vi "Get Pressure.vi"(6 "Channel":i32, 8 "error in (no error)":errorcluster, 11 "Instrument.Cryostat in":refnum<class "Instrument.Cryostat.lvclass">) -> (0 "error out":errorcluster, 1 "Status":string, 2 "Pressure (mbar)":dbl, 3 "Instrument.Cryostat out":refnum<class "Instrument.Cryostat.lvclass">)   [LabVIEW 2019, in "Instrument.Cryostat.lvclass"]
uses:
  Instrument.Cryostat.lvclass
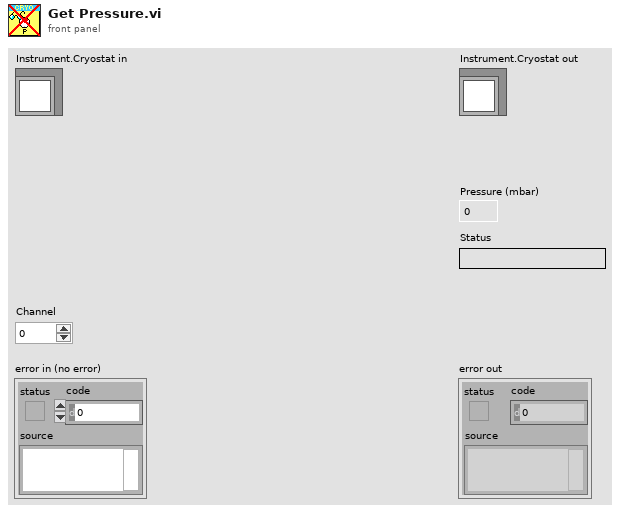
[diagram p1: front panel]
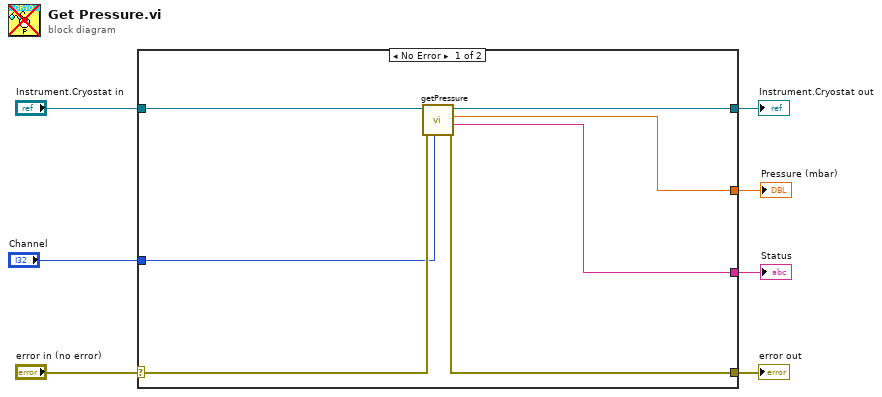
[diagram p0: block diagram]
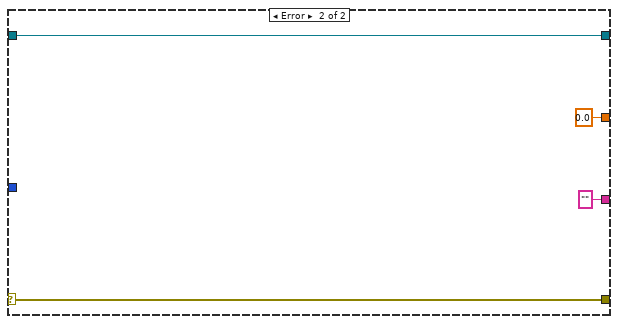
[diagram p2: hidden frame]
diagram:
  n1 = case shown="No Error" "error in (no error)" {
    selector: "error in (no error)" -> [w12 w18]
    tunnel: [w11 w18] -> w6
    tunnel: [w14 w17] -> w4
    tunnel: "Instrument.Cryostat in" -> [w13 w17]
    tunnel: [w10 "" ("Status")] -> w3
    tunnel: [w9 0.0 ("Pressure (mbar)")] -> w2
    tunnel: "Channel" -> [w8 _]
    frame No Error {
      n2 = call-dynamic "getPressure.vi"("Channel"=w8, "error in (no error)"=w12, "Instrument.Cryostat in"=w13) -> ("error out"=w11:errorcluster, "Status"=w10:string, "Pressure (mbar)"=w9:dbl, "Instrument.Cryostat out"=w14:refnum<class "Instrument.Cryostat.lvclass">)  [unwired: 5 in]
    }
    frame Error {
    }
  }
  "error out" <- w6
  "Instrument.Cryostat out" <- w4
  "Pressure (mbar)" <- w2
  "Status" <- w3
